vi "QuickProfile.vi"(7 "Image IN":sgl[][](array[numeric]), 11 "Pixel Size (nm)":dbl, 13 "Test Image":bool) -> ()   [LabVIEW 2012]
uses:
  <vilib>/Utility/file.llb/Write To Spreadsheet File (DBL).vi
panel:
  out "Lorentzian Measured FWHM (nm)":dbl
  out "Gaussian Measured 1/e Y (nm)":dbl
  out "Gaussian Measured 1/e X (nm)":dbl
  in  "Save ROI":bool
  in  "Power (%)":dbl
  in  "Delay (ps)":dbl
  out "Lorentzian Fit Width (nm)":dbl
  out "Gaussian Fit Width Y (nm)":dbl
  out "Gaussian Fit Width X (nm)":dbl
  in  "Auto Save":bool
  in  "Save Data":bool
  in  "Save File":path
  out "Constant Y Slice":cluster{"X Values":dbl[], sgl[]}[](graph)
  out "Constant X Slice":cluster{"X Values":dbl[], sgl[]}[](graph)
  in  "Fit ROI":bool
  out "Gaussian Fit":dbl[][](graph)
  out "Lorentzian Fit":dbl[][](graph)
  out "Current ROI":sgl[][](graph)
  in  "Region Size (px)":dbl=60.0
  in  "Quit":bool
  out "Image Display":sgl[][](graph)
  # "Constant Y"
  # "Constant X"
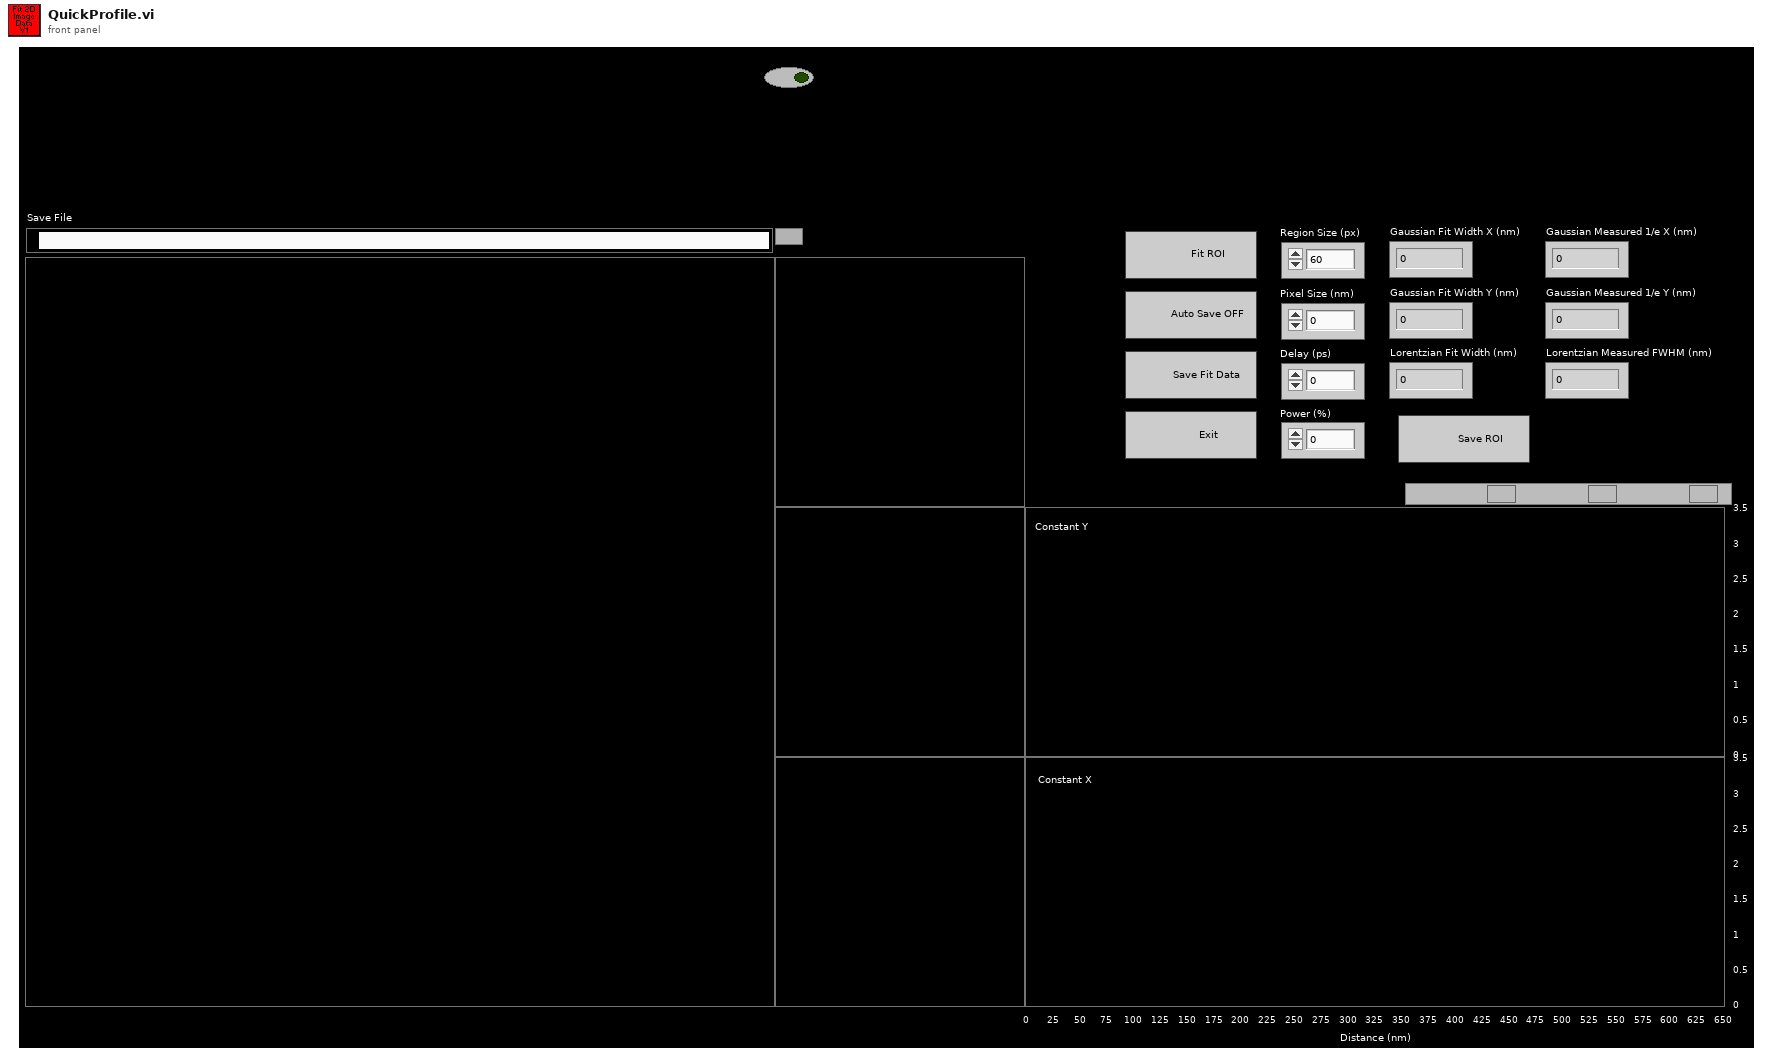
[diagram p1: front panel]
types:
  T1 = enum16{"open", "replace", "create", "open or create", "replace or create", "replace or create with confirmation"}
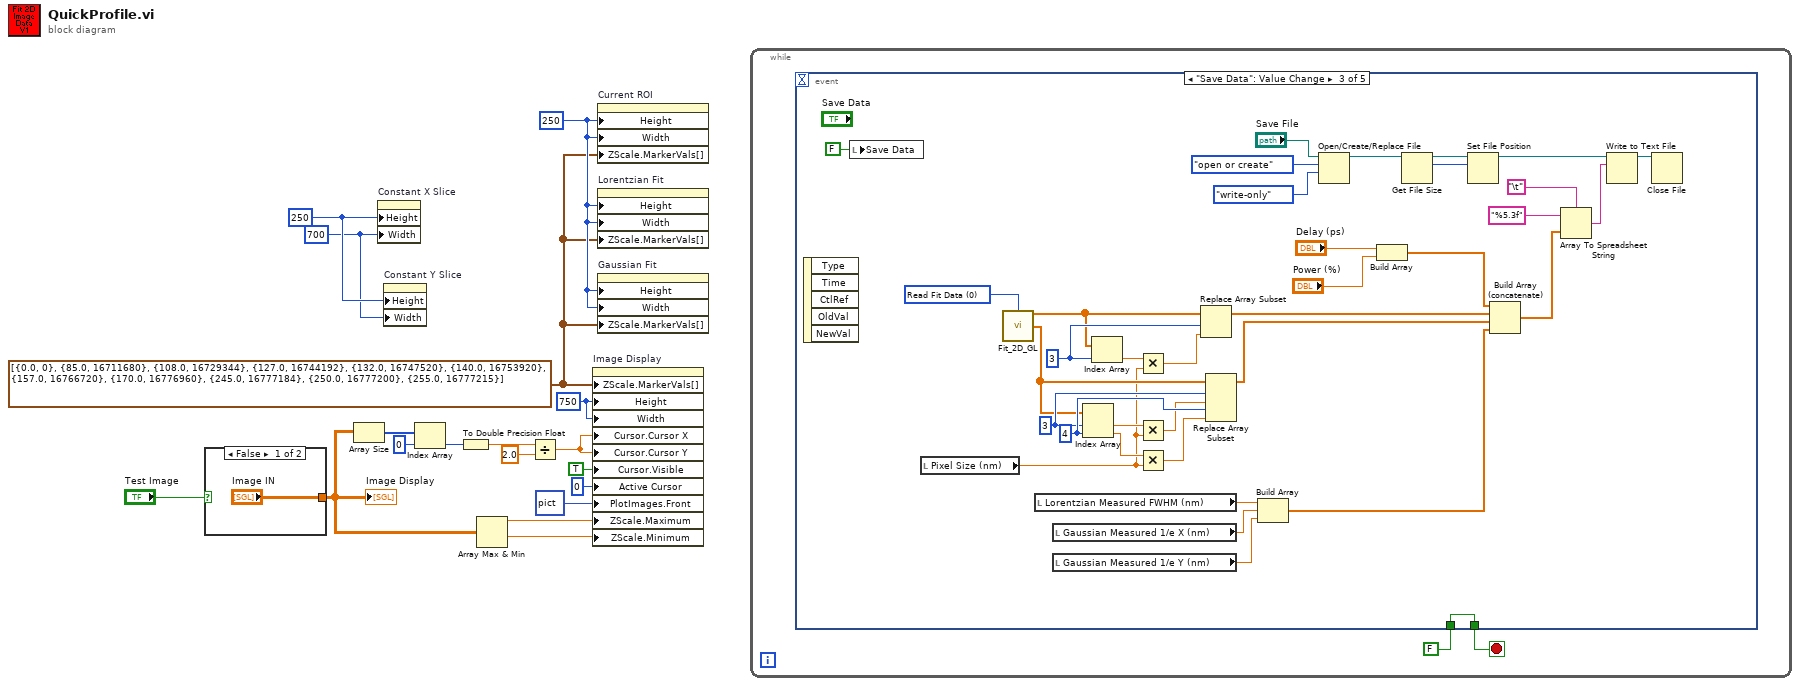
[diagram p0: block diagram]
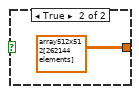
[diagram p2: hidden frame]
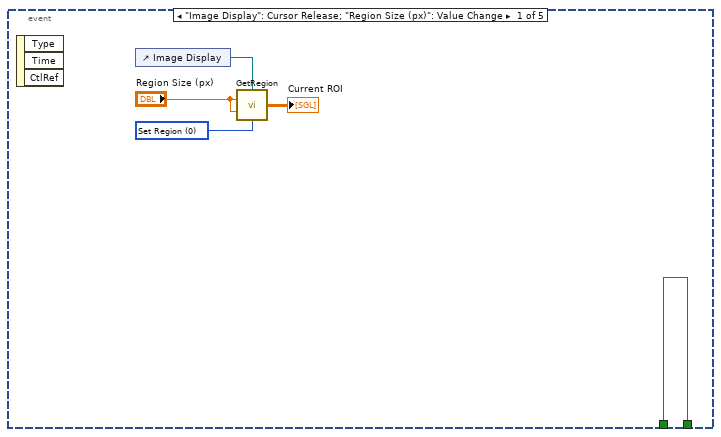
[diagram p3: hidden frame]
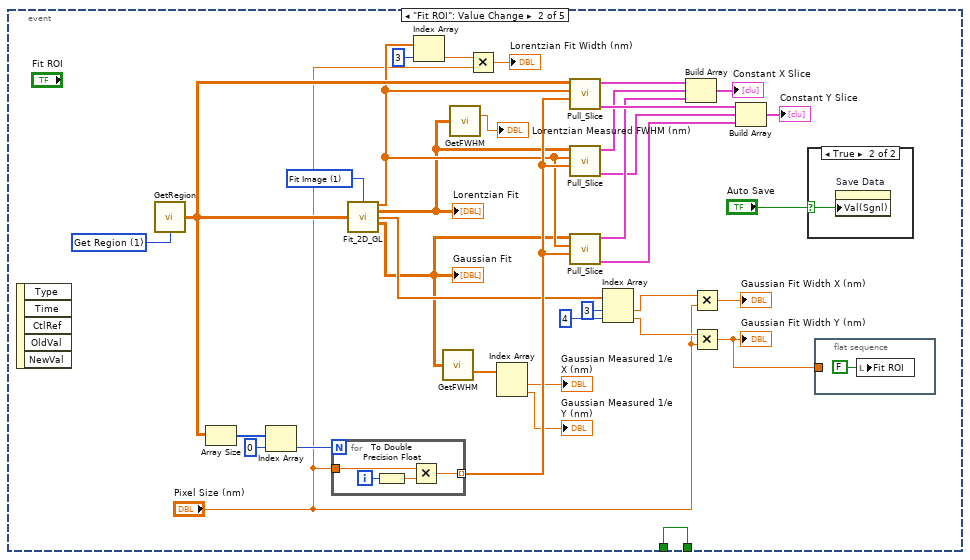
[diagram p4: hidden frame]
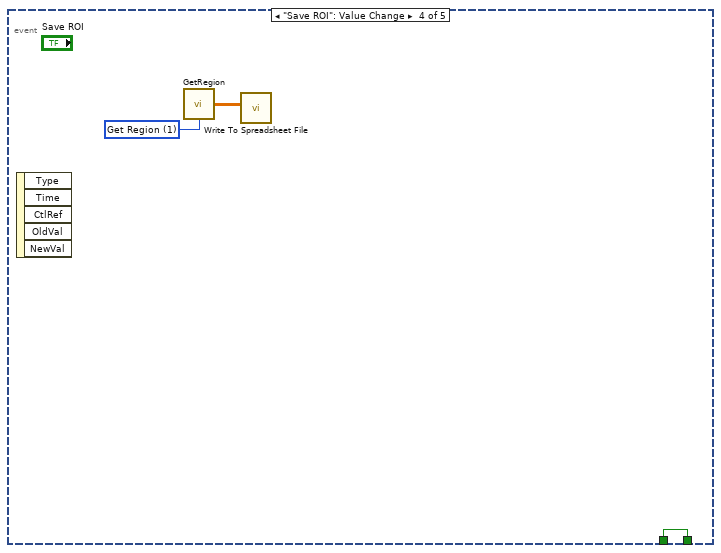
[diagram p6: hidden frame]
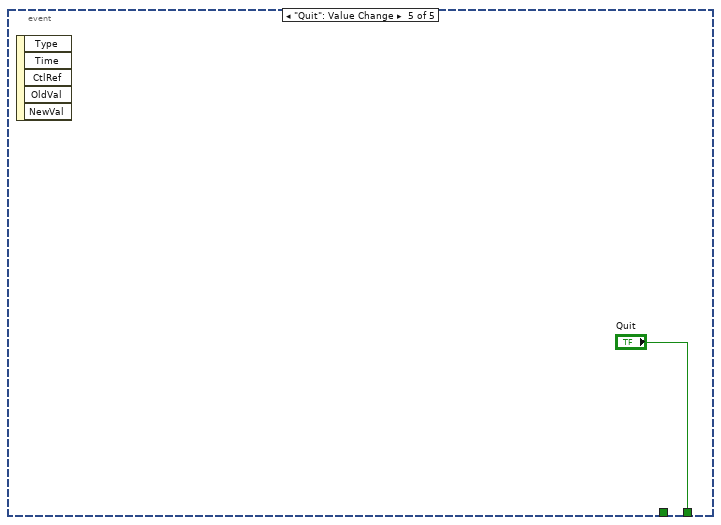
[diagram p7: hidden frame]
diagram:
  w11 = u32 700 ("Plot Area:Size:Width")
  w12 = u32 250 ("Plot Area:Size:Height")
  w14 = u32 250 ("Plot Area:Size:Height")
  w18 = u32 750 ("Plot Area:Size:Height")
  w13 = cluster{dbl, u32}[] [{0.0, 0}, {85.0, 16711680}, {108.0, 16729344}, {127.0, 16744192}, {132.0, 16747520}, {140.0, 16753920}, {157.0, 16766720}, {170.0, 16776960}, {245.0, 16777184}, {250.0, 16777200}, {255.0, 16777215}] ("Z Scale.Marker Values[]")
  n1 = case shown="False" "Test Image" {
    tunnel: ["Image IN" sgl[][] array512x512[262144 elements] ("Im Prev")] -> w7
    frame False {
    }
    frame True {
    }
  }
  "Image Display" <- w7
  n2 = Array Size(array=w7) -> (size(s)=w6:i32[])
  n3 = property on="Constant X Slice" class="XYGraph (strict)"("Height"=w12, "Width"=w11) -> ()  [unwired: 2 in, 2 out]
  n4 = property on="Constant Y Slice" class="XYGraph (strict)"("Height"=w12, "Width"=w11) -> ()  [unwired: 2 in, 2 out]
  n5 = Index Array(array=w6, index=0) -> (element=w4:i32)
  n6 = To Double Precision Float(number=w4) -> (double precision float=w2:dbl)
  n7 = Array Max & Min(array=w7) -> (max value=w10:sgl, min value=w9:sgl)  [unwired: 2 out]
  n8 = Divide(x=w2, y=2.0) -> (x/y=w1:dbl)
  n9 = property on="Image Display" class="IntGraph (strict)"("ZScale.MarkerVals[]"=w13, "Height"=w18, "Width"=w18, "Cursor.Cursor X"=w1, "Cursor.Cursor Y"=w1, "Cursor.Visible"=TRUE, "Active Cursor"=u32 0, "PlotImages.Front"=picture data[5B] ("Plot Images:Front"), "ZScale.Maximum"=w10, "ZScale.Minimum"=w9) -> ()  [unwired: 2 in, 2 out]
  n10 = property on="Current ROI" class="IntGraph (strict)"("Height"=w14, "Width"=w14, "ZScale.MarkerVals[]"=w13) -> ()  [unwired: 2 in, 2 out]
  n11 = property on="Lorentzian Fit" class="IntGraph (strict)"("Height"=w14, "Width"=w14, "ZScale.MarkerVals[]"=w13) -> ()  [unwired: 2 in, 2 out]
  n12 = property on="Gaussian Fit" class="IntGraph (strict)"("Height"=w14, "Width"=w14, "ZScale.MarkerVals[]"=w13) -> ()  [unwired: 2 in, 2 out]
  n13 = while {
    stop <- w22 stop-if-true
    n14 = event shown="[2] \"Save Data\": Value Change" {
      selector: _ -> [_ _ _ _ _]
      dyn-events: _ -> [_ _ _ _ _]
      timeout: _ -> [_ _ _ _ _]
      tunnel: [w26 w62 w100 w106 "Quit"] -> w22
      tunnel: FALSE -> [w26 w62 w100 w106 _]
      event "Image Display": Cursor Release; "Region Size (px)": Value Change {
        w24 = u16 0 items=["Set Region", "Get Region"] ("Action")
        n15 = event-data() -> ()  [unwired: 1 in, 3 out]
        n16 = control-ref of="Image Display"() -> (w27:refnum<vi>)
        n17 = call "GetRegion.vi"("IntGraph REF"=w27, "Y Width (PX)"="Region Size (px)", "X Width (PX)"="Region Size (px)", "Action"=w24) -> ("Region Out"=→"Current ROI":sgl[][])  [unwired: 11 in]
      }
      event "Fit ROI": Value Change {
        w60 = u16 1 items=["Read Fit Data", "Fit Image"] ("Action")
        w61 = u16 1 items=["Set Region", "Get Region"] ("Action")
        n18 = event-data() -> ()  [unwired: 1 in, 5 out]
        n19 = call "GetRegion.vi"("Action"=w61) -> ("Region Out"=w50:sgl[][])  [unwired: 14 in]
        n20 = Array Size(array=w50) -> (size(s)=w59:i32[])
        n21 = Index Array(array=w59, index=0) -> (element=w57:i32)
        n22 = for {
          N: w57 -> [_]
          tunnel: "Pixel Size (nm)" -> [w67]
          tunnel: [w65] -> w56 mode=indexing
          i -> [w68]
          n23 = To Double Precision Float(number=w68) -> (double precision float=w66:dbl)
          n24 = Multiply(x=w67, y=w66) -> (x*y=w65:dbl)
        }
        n25 = call "Fit_2D_GL.vi"("Action"=w60, "Image IN"=w50) -> ("Lorentz Fit Parameters"=w45:dbl[], "Lorentzian Image"=w33:dbl[][], "Gaussian Fit Parameters"=w47:dbl[], "Gaussian Image"=w32:dbl[][])  [unwired: 9 in, 1 out]
        "Gaussian Fit" <- w32
        "Lorentzian Fit" <- w33
        n26 = Index Array(array=w45, index=3) -> (element=w40:dbl)
        n27 = call "GetFWHM.vi"("Image IN"=w32) -> ("1/e Diameter (x and y)"=w31:dbl[])  [unwired: 13 in, 1 out]
        n28 = call "GetFWHM.vi"("Image IN"=w33) -> ("FWHM"=→"Lorentzian Measured FWHM (nm)":dbl)  [unwired: 13 in, 1 out]
        n29 = Multiply(x=w40, y="Pixel Size (nm)") -> (x*y=→"Lorentzian Fit Width (nm)":dbl)
        n30 = Index Array(array=w31) -> (element #1=→"Gaussian Measured 1/e X (nm)":dbl, element #2=→"Gaussian Measured 1/e Y (nm)":dbl)  [unwired: 2 in]
        n31 = call "Pull_Slice.vi"("X Values"=w56, "Fit Parameters"=w45, "ROI Image"=w50) -> ("Constant X Slice"=w55:cluster{"X Values":dbl[], sgl[]}, "Constant Y Slice"=w41:cluster{"X Values":dbl[], sgl[]})  [unwired: 7 in]
        n32 = call "Pull_Slice.vi"("X Values"=w56, "Fit Parameters"=w45, "ROI Image"=w33) -> ("Constant X Slice"=w52:cluster{"X Values":dbl[], sgl[]}, "Constant Y Slice"=w54:cluster{"X Values":dbl[], sgl[]})  [unwired: 7 in]
        n33 = call "Pull_Slice.vi"("X Values"=w56, "Fit Parameters"=w45, "ROI Image"=w32) -> ("Constant X Slice"=w51:cluster{"X Values":dbl[], sgl[]}, "Constant Y Slice"=w53:cluster{"X Values":dbl[], sgl[]})  [unwired: 7 in]
        n34 = Index Array(array=w47, index #1=3 ("index"), index #2=4 ("index")) -> (element #1=w38:dbl, element #2=w36:dbl)
        n35 = Build Array(w41, w54, w53) -> (→"Constant X Slice":cluster{"X Values":dbl[], sgl[]}[])
        n36 = Multiply(x=w38, y="Pixel Size (nm)") -> (x*y=→"Gaussian Fit Width X (nm)":dbl)
        n37 = Multiply(x=w36, y="Pixel Size (nm)") -> (x*y=w34:dbl)
        "Gaussian Fit Width Y (nm)" <- w34
        n38 = Build Array(w55, w52, w51) -> (→"Constant Y Slice":cluster{"X Values":dbl[], sgl[]}[])
        n39 = case shown="True" "Auto Save" {
          selector: "Auto Save" -> [_ w64]
          frame False {
          }
          frame True {
            n40 = property on="Save Data" class="Bool (strict)"("Val(Sgnl)"=w64) -> ()  [unwired: 2 in, 2 out]
          }
        }
        n41 = flat-sequence {
          tunnel: w34 -> [_]
          frame #0 {
            n42 = local write "Fit ROI"(FALSE ("Fit ROI")) -> ()
          }
        }
      }
      event "Save Data": Value Change {
        w87 = 4 ("index")
        w86 = 3 ("index")
        w78 = 3 ("index")
        w76 = u16 0 items=["Read Fit Data", "Fit Image"] ("Action")
        n43 = event-data() -> ()  [unwired: 1 in, 5 out]
        n44 = local write "Save Data"(FALSE ("Save Data")) -> ()
        n45 = local read "Pixel Size (nm)"() -> (w73:dbl)
        n46 = call "Fit_2D_GL.vi"("Action"=w76) -> ("Lorentz Fit Parameters"=w77:dbl[], "Gaussian Fit Parameters"=w81:dbl[])  [unwired: 10 in, 3 out]
        n47 = local read "Lorentzian Measured FWHM (nm)"() -> (w70:dbl)
        n48 = local read "Gaussian Measured 1/e X (nm)"() -> (w71:dbl)
        n49 = local read "Gaussian Measured 1/e Y (nm)"() -> (w72:dbl)
        n50 = Index Array(array=w81, index #1=w86, index #2=w87) -> (element #1=w82:dbl, element #2=w83:dbl)
        n51 = Index Array(array=w77, index=w78) -> (element=w79:dbl)
        n52 = Multiply(x=w79, y=w73) -> (x*y=w80:dbl)
        n53 = Multiply(x=w82, y=w73) -> (x*y=w84:dbl)
        n54 = Multiply(x=w83, y=w73) -> (x*y=w85:dbl)
        n55 = Replace Array Subset(array=w77, new element=w80, index=w78) -> (w75:dbl[])
        n56 = Replace Array Subset(array=w81, new element #1=w84, index #1=w86, new element #2=w85, index #2=w87) -> (w74:dbl[])
        n57 = Build Array(w70, w71, w72) -> (w69:dbl[])
        n58 = Open/Create/Replace File(file path (use dialog)="Save File", operation (0:open)=T1."open or create", access (0:read/write)=enum16{"read/write", "read-only", "write-only"}."write-only") -> (refnum out=w97:refnum<file>)  [unwired: 3 in, 2 out]
        n59 = Build Array("Delay (ps)", "Power (%)") -> (w88:dbl[])
        n60 = Get File Size(file=w97) -> (refnum out=w96:refnum<file>, size (in bytes)=w98:i64)  [unwired: 1 in, 1 out]
        n61 = Set File Position(offset (in bytes) (0)=w98, refnum=w96) -> (refnum out=w99:refnum<file>)  [unwired: 2 in, 1 out]
        n62 = Build Array (concatenate)(w88, w75, w74, w69) -> (w91:dbl[])
        n63 = Array To Spreadsheet String(delimiter (Tab)="\t", array=w91, 3:"%5.3f" ("format string")) -> (spreadsheet string=w93:string)
        n64 = Write to Text File(file (use dialog)=w99, text=w93) -> (refnum out=w101:refnum<file>)  [unwired: 2 in, 2 out]
        n65 = Close File(refnum=w101) -> ()  [unwired: 1 in, 2 out]
      }
      event "Save ROI": Value Change {
        w107 = u16 1 items=["Set Region", "Get Region"] ("Action")
        n66 = event-data() -> ()  [unwired: 1 in, 5 out]
        n67 = call "GetRegion.vi"("Action"=w107) -> ("Region Out"=w105:sgl[][])  [unwired: 14 in]
        n68 = call-poly <vilib>:"Write To Spreadsheet File.vi"("2D data"=w105) -> ()  [unwired: 7 in, 1 out]
      }
      event "Quit": Value Change {
        n69 = event-data() -> ()  [unwired: 1 in, 5 out]
      }
    }
  }
